vi "compass_calibrate.vi"   [LabVIEW 2012, in "Mecanum Drive.lvrbt"]
uses:
  Mecanum Drive.lvrbt
  SubVIs/auto_drive_TYP.ctl
  <vilib>/NXT/Block Support/NXT_InputPort.ctl
types:
  T1 = typedef "NXT_InputPort.ctl" = u32
  T2 = typedef "auto_drive_TYP.ctl" = cluster{"Left X":i8, "Left Y":i8, "Right X":i8, "Power (100)":i8, "Wait (ms)":u32, "Enc/Deg Target":i32, "Move Type":enum16{"Relative Degrees", "Wait", "Encoder"}}
  T3 = typedef "LVHSConnector.ctl" = refnum<class "BrickReference.lvclass">
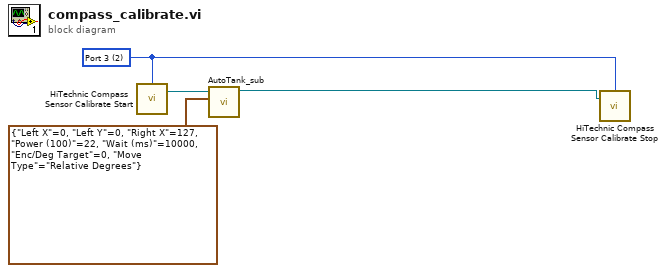
[diagram p0: block diagram]
diagram:
  w1 = T1 2 items=["Port 1", "Port 2", "Port 3", "Port 4"] ("Port")
  n1 = call <vilib>:"HiTechnic Compass Sensor Calibrate Start.vi"("Port"=w1) -> ("NXT/EV3"=w4:T3)  [unwired: 3 in]
  n2 = call "AutoTank_sub.vi"("Drive Control"=T2 {"Left X"=0, "Left Y"=0, "Right X"=127, "Power (100)"=22, "Wait (ms)"=10000, "Enc/Deg Target"=0, "Move Type"=enum."Relative Degrees"}, "NXT/EV3"=w4) -> ("NXT/EV3 out"=w3:T3)  [unwired: 8 in, 1 out]
  n3 = call <vilib>:"HiTechnic Compass Sensor Calibrate Stop.vi"("NXT/EV3"=w3, "Port"=w1) -> ()  [unwired: 1 in, 2 out]
